vi "test timer.vi"() -> ()   [LabVIEW 2015]
panel:
  out "millisecond timer value":u32
  in  "Stop Button":bool
  in  "millisecond multiple":u32
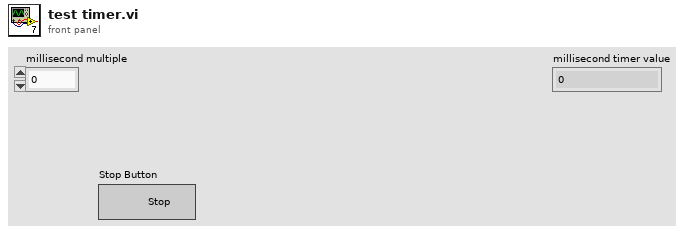
[diagram p1: front panel]
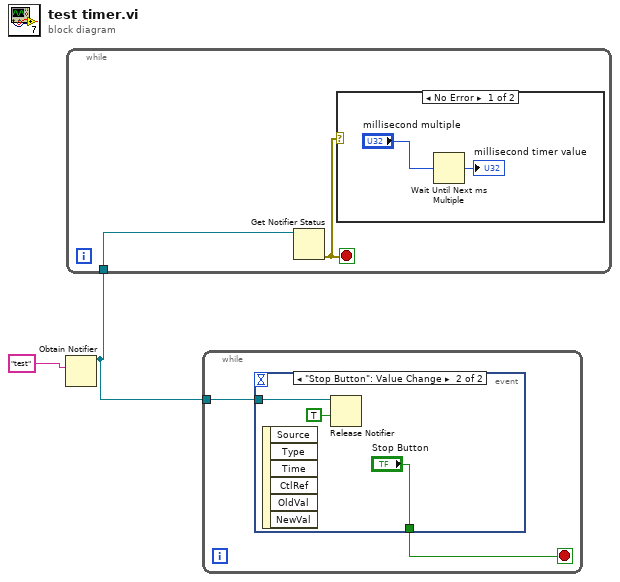
[diagram p0: block diagram]
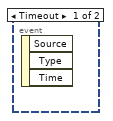
[diagram p2: hidden frame]
diagram:
  n1 = Obtain Notifier(notification data type="test") -> (notifier out=w1:refnum<notifier>)  [unwired: 3 in, 2 out]
  n2 = while {
    tunnel: w1 -> [w3]
    stop <- w4 stop-if-true
    n3 = Get Notifier Status(notifier=w3) -> (error out=w4:errorcluster)  [unwired: 1 in, 4 out]
    n4 = case shown="No Error" w4 {
      frame No Error {
        n5 = Wait Until Next ms Multiple(millisecond multiple="millisecond multiple") -> (millisecond timer value=→"millisecond timer value":u32)
      }
      frame Error {
      }
    }
  }
  n6 = while {
    tunnel: w1 -> [w7]
    stop <- w8 stop-if-true
    n7 = event shown="[1] \"Stop Button\": Value Change" {
      selector: _ -> [_ _]
      dyn-events: _ -> [_ _]
      timeout: _ -> [_ _]
      tunnel: [_ "Stop Button"] -> w8
      tunnel: w7 -> [_ w10]
      event Timeout {
        n8 = event-data() -> ()  [unwired: 1 in, 3 out]
      }
      event "Stop Button": Value Change {
        n9 = event-data() -> ()  [unwired: 1 in, 6 out]
        n10 = Release Notifier(notifier=w10, force destroy? (F)=TRUE) -> ()  [unwired: 1 in, 3 out]
      }
    }
  }
